vi "Enumerate AO Endpoints.vi"(8 "error in (no error)":errorcluster, 11 "Tosca in":refnum<class "Parameters.lvclass">) -> (0 "error out":errorcluster, 2 "Endpoints":string[](array[string]), 3 "Tosca out":refnum<class "Parameters.lvclass">)   [LabVIEW 2020, in "Parameters.lvclass"]
uses:
  Parameters.lvclass
  Parameters.lvclass/Parameters.ctl
  State/State.lvclass/State.ctl
  State/Read SigMan.vi
  epl-vi-lib/Signal Synthesis VIs/4th Generation/Classes/SignalManager/SignalManager.lvclass
  State/State.lvclass
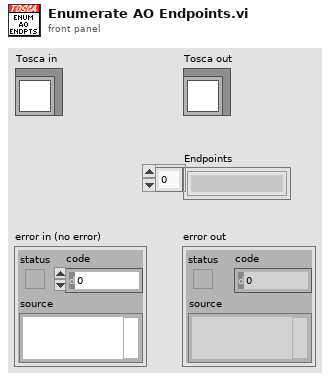
[diagram p1: front panel]
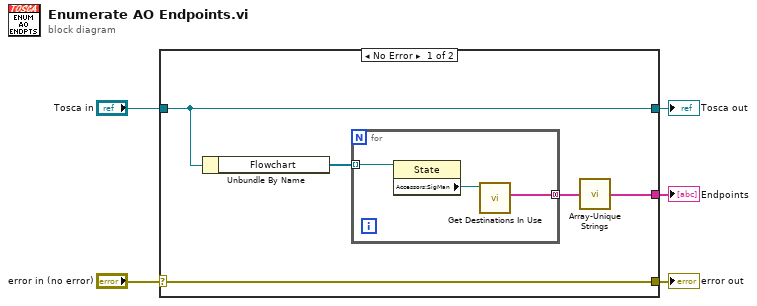
[diagram p0: block diagram]
diagram:
  n1 = case shown="No Error" "error in (no error)" {
    selector: "error in (no error)" -> [w10 w15]
    tunnel: [w10 w15] -> w4
    tunnel: [w9 w14] -> w2
    tunnel: "Tosca in" -> [w9 w14]
    tunnel: [w6 _] -> w1
    frame No Error {
      n2 = Unbundle By Name(w9) -> ("Flowchart"=w8:refnum<class "State.lvclass">[])
      n3 = for {
        tunnel: w8 -> [w13] mode=indexing
        tunnel: [w11] -> w7 mode=concatenating
        n4 = property class="State"(reference=w13) -> ("Accessors:SigMan"=w12:refnum<class "SignalManager.lvclass">)  [unwired: 1 in, 2 out]
        n5 = call "Get Destinations In Use.vi"("SigMan in"=w12) -> ("Destinations in use"=w11:string[])  [unwired: 8 in, 2 out]
      }
      n6 = call "Array-Unique Strings.vi"("Strings"=w7) -> ("Unique strings"=w6:string[])  [unwired: 4 in]
    }
    frame Error {
    }
  }
  "error out" <- w4
  "Tosca out" <- w2
  "Endpoints" <- w1
